vi "Set Server State Ref.vi"(10 "Server Internal State Ref":refnum<data-value>, 11 "Template Server in":refnum<class "MeasurementService_Template.lvclass">) -> (3 "Template Server out":refnum<class "MeasurementService_Template.lvclass">)   [LabVIEW 2020, in "MeasurementService_Template.lvlib" / "MeasurementService_Template.lvclass"]
uses:
  MeasurementService_Template.lvclass
  typeDefs/Server State Data.ctl
  MeasurementService_Template.lvclass/MeasurementService_Template.ctl
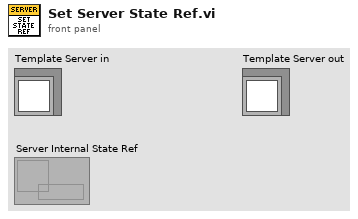
[diagram p1: front panel]
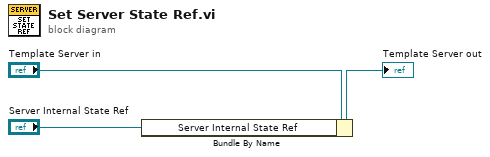
[diagram p0: block diagram]
diagram:
  n1 = Bundle By Name(cluster="Template Server in", "Server Internal State Ref"="Server Internal State Ref") -> (→"Template Server out":refnum<class "MeasurementService_Template.lvclass">)
